vi "DATA_ACQUISITION.vi"(2 "error in":errorcluster, 3 "SAMPLING FREQ":dbl format="%0.2f", 4 "# SAMPLES":i32, 5 "DAQ CHANNEL":tag) -> (0 "error out":errorcluster, 1 "data":waveform(dbl))   [LabVIEW 2023]
uses:
  <vilib>/DAQmx/read.llb/DAQmx Read (Analog Wfm 1Chan NSamp).vi
  <vilib>/DAQmx/create/channels.llb/DAQmx Create Channel (AI-Voltage-Basic).vi
  <vilib>/DAQmx/configure/timing.llb/DAQmx Timing (Sample Clock).vi
  <vilib>/DAQmx/miscellaneous.llb/DAQmx Fill In Error Info.vi
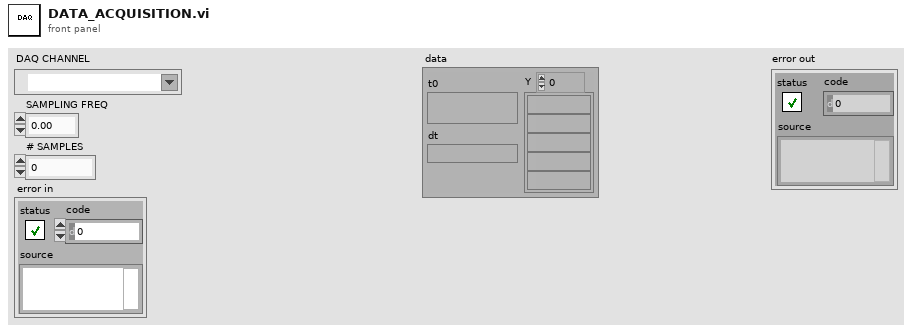
[diagram p1: front panel]
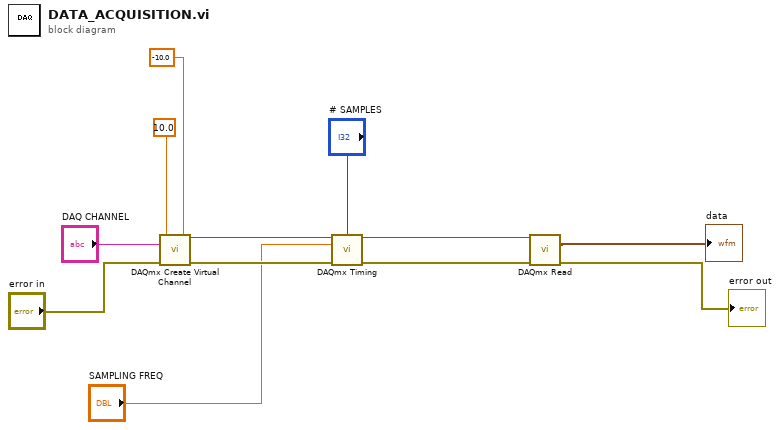
[diagram p0: block diagram]
diagram:
  n1 = call-poly <vilib>:"DAQmx Create Virtual Channel.vi"("maximum value"=10.0, "minimum value"=-10.0, "physical channels"="DAQ CHANNEL", "error in"="error in") -> ("task out"=w12:refnum<k21>, "error out"=w11:errorcluster)  [unwired: 10 in]
  n2 = call-poly <vilib>:"DAQmx Timing.vi"("task/channels in"=w12, "samples per channel"="# SAMPLES", "rate"="SAMPLING FREQ", "error in"=w11) -> ("task out"=w10:refnum<k21>, "error out"=w9:errorcluster)  [unwired: 10 in]
  n3 = call-poly <vilib>:"DAQmx Read.vi"("task/channels in"=w10, "error in"=w9) -> ("data"=→"data":waveform(dbl), "error out"=→"error out":errorcluster)  [unwired: 11 in, 1 out]
